vi "Day5.vi"(10 "UpdatedPages":string="75,47,61,53,29\n97,61,53,29,13\n75,29,13\n75,97,47,61,53\n61,13,29\n97,13,75,29,47", 11 "OrderingRules":string="47|53\n97|13\n97|61\n97|47\n75|29\n61|13\n75|53\n29|13\n97|29\n53|29\n61|53\n97|53\n61|29\n47|13\n75|47\n97|75\n47|61\n75|61\n47|29\n75|13\n53|13") -> (3 "Result":i64)   [LabVIEW 2024]
uses:
  <vilib>/Utility/miscctls.llb/LVMapReplaceAction.ctl
panel:
  out "MidNumbers":i64[](array[numeric])
  out "Good Lines":bool[](array[boolean])
  out "Map":map{i32, i32[]}(c390)
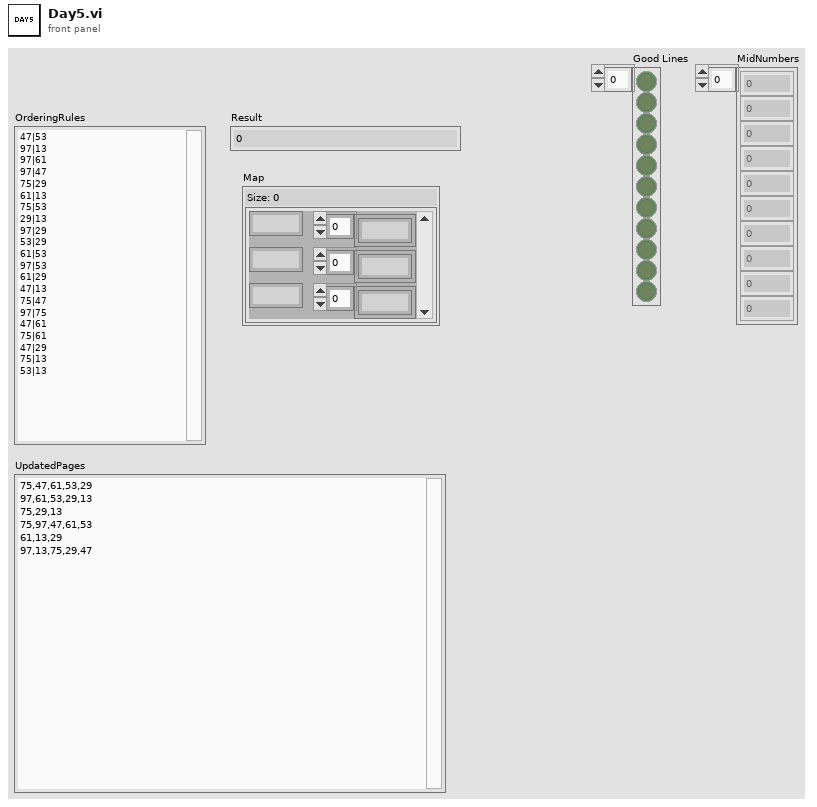
[diagram p1: front panel]
types:
  T1 = typedef "LVMapReplaceAction.ctl" = enum32{"Modify Entry only if found", "Add or Modify Entry", "Delete Entry"}
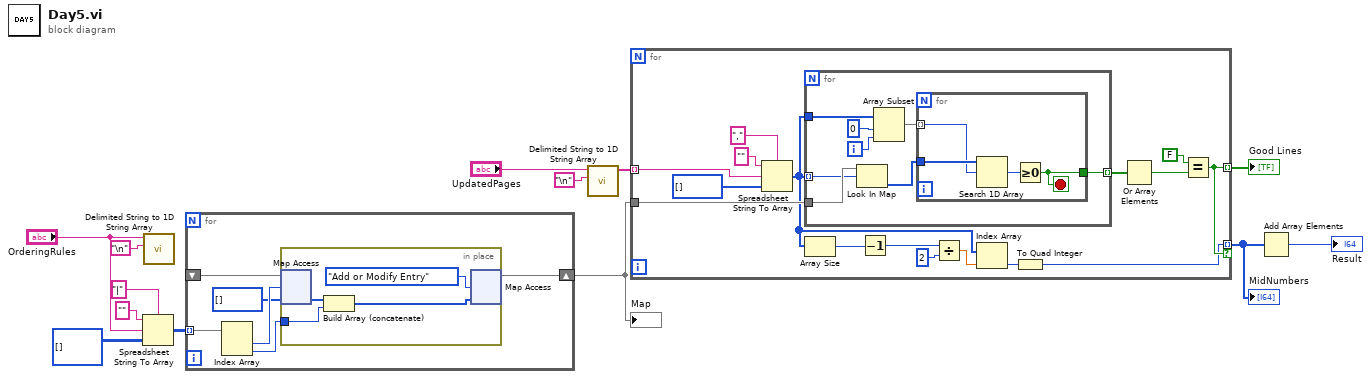
[diagram p0: block diagram]
diagram:
  n1 = Spreadsheet String To Array(delimiter (Tab)="|", format string="", spreadsheet string="OrderingRules", array type (2D Dbl)=i32[][] []) -> (array=w5:i32[][])
  n2 = call <vilib>:"Delimited String to 1D String Array.vi"("delimiter"="\n", "delimited string"="OrderingRules") -> ()  [unwired: 9 in, 1 out]
  n3 = for {
    tunnel: w5 -> [w19] mode=indexing
    shift-right: [w14] -> w4
    shift-left: _ -> [w17]
    n4 = Index Array(array=w19) -> (element #1=w18:i32, element #2=w15:i32)  [unwired: 2 in]
    n5 = in-place {
      in-place-border: w15 -> [w22]
      n6 = in-place-map #1(w17, w18, i32[] []) -> (w23:i32[])  [unwired: 1 out]
      n7 = Build Array (concatenate)(w23, w22) -> (w21:i32[])
      n8 = in-place-map #1(w21, LVMapReplaceAction."Add or Modify Entry" ("action")) -> (w14:map{i32, i32[]})  [unwired: 2 out]
    }
  }
  "Map" <- w4
  n9 = call <vilib>:"Delimited String to 1D String Array.vi"("delimiter"="\n", "delimited string"="UpdatedPages") -> ("string array"=w10:string[])  [unwired: 9 in]
  n10 = for {
    tunnel: w10 -> [w39] mode=indexing
    tunnel: w4 -> [w35]
    tunnel: [w26] -> w3 mode=indexing
    tunnel: [w24] -> w2 mode=indexing if=w26
    n11 = Spreadsheet String To Array(delimiter (Tab)=",", format string="", spreadsheet string=w39, array type (2D Dbl)=i32[] []) -> (array=w27:i32[])
    n12 = for {
      tunnel: w27 -> [w46] mode=indexing
      tunnel: w35 -> [w47]
      tunnel: w27 -> [w43]
      tunnel: [w40] -> w34 mode=indexing
      i -> [w45]
      n13 = Look In Map(map=w47, key=w46) -> (value=w41:i32[])  [unwired: 1 in, 1 out]
      n14 = Array Subset(array=w43, index=0, length=w45) -> (w42:i32[])
      n15 = for {
        tunnel: w42 -> [w50] mode=indexing
        tunnel: w41 -> [w51]
        tunnel: [w48] -> w40
        stop <- w48 stop-if-true
        n16 = Search 1D Array(1D array=w51, element=w50) -> (index of element=w49:i32)  [unwired: 1 in]
        n17 = Greater Or Equal To 0?(x=w49) -> (x >= 0?=w48:bool)
      }
    }
    n18 = Array Size(array=w27) -> (size(s)=w31:i32)
    n19 = Decrement(x=w31) -> (x-1=w30:i32)
    n20 = Divide(x=w30, y=2) -> (x/y=w28:dbl)
    n21 = Index Array(array=w27, index=w28) -> (element=w25:i32)
    n22 = To Quad Integer(1:w25) -> (0:w24:i64)
    n23 = Or Array Elements(Boolean array=w34) -> (logical OR=w33:bool)
    n24 = Equal?(x=FALSE, y=w33) -> (x = y?=w26:bool)
  }
  "Good Lines" <- w3
  "MidNumbers" <- w2
  n25 = Add Array Elements(numeric array=w2) -> (sum=→"Result":i64)
